vi "SCD41-string-array-to-data.vi"(9 "Starting Index":i32, 11 "Data In (string array)":string[](array[string])) -> (0 "SCD41: data output":T1 {"Humidity (%)" format="%.2f"; "Temp (degC)" format="%.2f"; "CO2 (ppm)" format="%.2f"}, 1 "SCD41: Humidity (%)":dbl format="%.2f", 2 "SCD41: Temp (degC)":dbl format="%.2f", 3 "SCD41: CO2 (ppm)":dbl format="%.2f")   [LabVIEW 2021]
uses:
  SCD41.ctl
panel:
  out "CD1: Humidity":string
  out "SCD41: Temp":string
  out "SCD41: CO2":string
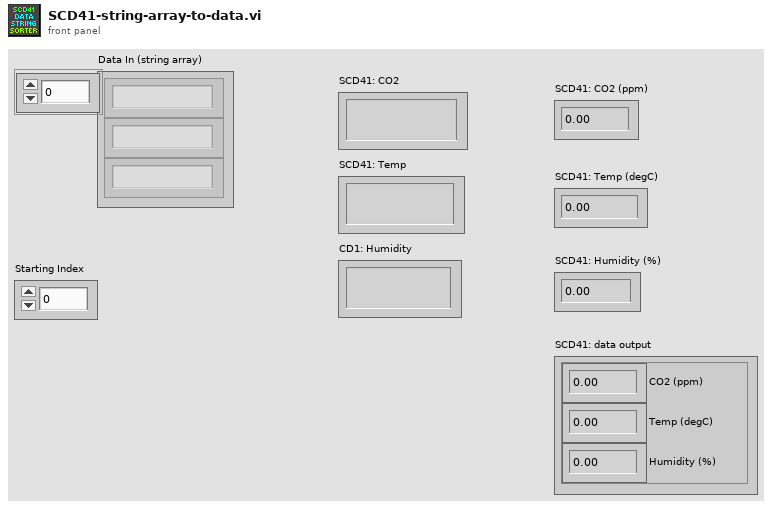
[diagram p1: front panel]
types:
  T1 = typedef "SCD41.ctl" = cluster{"CO2 (ppm)":dbl, "Temp (degC)":dbl, "Humidity (%)":dbl}
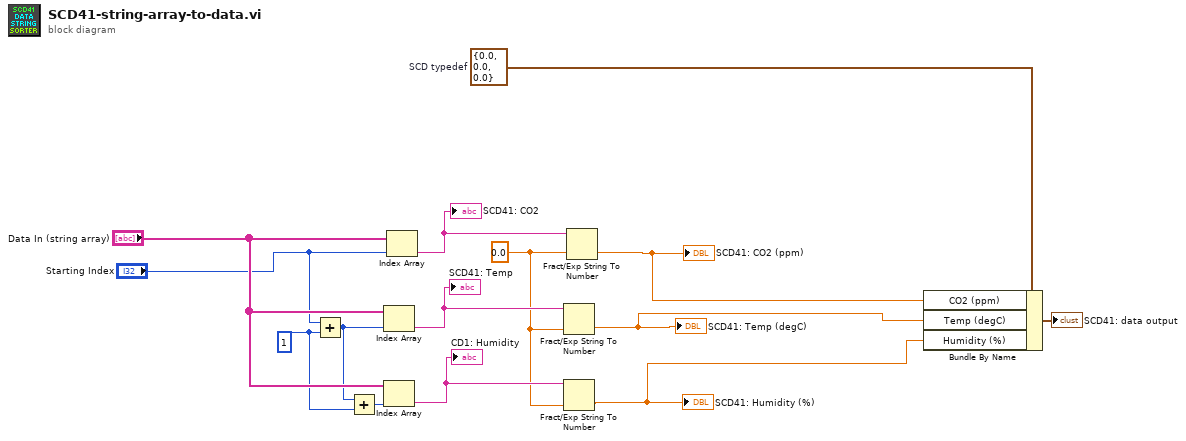
[diagram p0: block diagram]
diagram:
  w5 = T1 {"CO2 (ppm)"=0.0, "Temp (degC)"=0.0, "Humidity (%)"=0.0}  # SCD typedef
  w10 = 1 ("y")
  w6 = 0.0
  n1 = Add(x="Starting Index", y=w10) -> (x+y=w11:i32)
  n2 = Add(x=w11, y=w10) -> (x+y=w12:i32)
  n3 = Index Array(array="Data In (string array)", index=w11) -> (element=w9:string)
  "SCD41: Temp" <- w9
  n4 = Index Array(array="Data In (string array)", index=w12) -> (element=w7:string)
  "CD1: Humidity" <- w7
  n5 = Index Array "Index Array"(array="Data In (string array)", index="Starting Index") -> (element=w8:string)
  "SCD41: CO2" <- w8
  n6 = Fract/Exp String To Number(string=w9, default (0 dbl)=w6) -> (number=w3:dbl)  [unwired: 2 in, 1 out]
  "SCD41: Temp (degC)" <- w3
  n7 = Fract/Exp String To Number(string=w7, default (0 dbl)=w6) -> (number=w2:dbl)  [unwired: 2 in, 1 out]
  "SCD41: Humidity (%)" <- w2
  n8 = Fract/Exp String To Number(string=w8, default (0 dbl)=w6) -> (number=w4:dbl)  [unwired: 2 in, 1 out]
  "SCD41: CO2 (ppm)" <- w4
  n9 = Bundle By Name(cluster=w5, "CO2 (ppm)"=w4, "Temp (degC)"=w3, "Humidity (%)"=w2) -> (→"SCD41: data output":T1)
